vi "Step Response - Air Heater.vi"() -> ()   [LabVIEW 2021]
uses:
  <vilib>/Simulation/Scripting/Companion Diagram/SimConfigNode/SimParams.ctl
  <vilib>/Simulation/Scripting/Companion Diagram/SimConfigNode/_simSolvers.ctl
  <vilib>/Simulation/Implementation/Shared/SIMSCR Execution Mode.ctl
  <vilib>/Simulation/Param Hierarchy/Typedefs/SIMPH Param Control Actions.ctl
  <vilib>/Simulation/Implementation/Shared/NILVSim_ParamChanged.vi
  <vilib>/Simulation/Implementation/Shared/NILVSIM_BeginStep.vi
  <vilib>/Simulation/Implementation/Shared/NILVSim_Manager.vi
  <vilib>/Utility/error.llb/Clear Errors.vi
  <vilib>/Simulation/Implementation/Shared/NILVSim_FinalizeModel.vi
  <vilib>/Simulation/Implementation/Shared/SIM Unbundle Sim Info.vi
  <vilib>/Simulation/Implementation/Shared/NILVSim_Initialize.vi
  <vilib>/Simulation/Utility/Implementation/NILVSim Get Time and IsAcceptedStep.vi
  <vilib>/Simulation/Implementation/Shared/SIMSH Read Queue.vi
  <vilib>/Simulation/Implementation/Shared/NILVSim_GetModelError.vi
  <vilib>/Simulation/Implementation/Shared/SIM Bundle Sim Info.vi
  <vilib>/Simulation/Implementation/XNodeFramework/SimXNode/SimX.xnode
  Model - Air Heater.vi
  <vilib>/Simulation/Scripting/Companion Diagram/SimConfigNode/SimDog.xnode
  <vilib>/Simulation/Implementation/Shared/NI_SIM_Implementation.lvlib
panel:
  in  "T_init [C]":dbl
  in  "T [s]":dbl
  in  "T_delay [s]":dbl
  in  "T_env [C]":dbl
  in  "K [C/V]":dbl
  in  "u [V]":dbl
  in  "Time Step [s]":dbl
  in  "stop":bool
  out "Control chart":dbl(graph)
  out "Temperature Chart":dbl(graph)
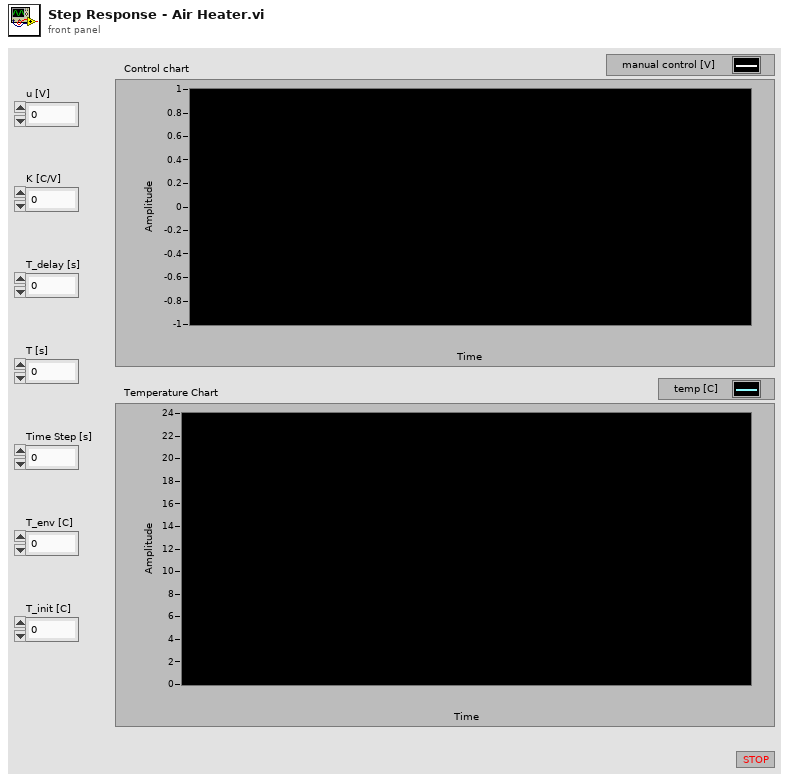
[diagram p1: front panel]
types:
  T1 = enum16{"Simulate to Completion", "Single Time-Step Simulation (Fixed Step Only)"}
  T2 = typedef "SIMSCR Execution Mode.ctl" = enum16{"Simulate to Completion", "Single Time-Step Simulation (Fixed Step Only)"}
  T3 = typedef "SIMPH Param Control Actions.ctl" = enum16{"get params", "set params"}
  T4 = cluster{"SIMSH Sim Time":dbl, "lower limit":dbl, "Divide":cluster{"x/y":dbl}, "Subtract":cluster{"x-y":dbl}, "Transport Delay":cluster{"output":dbl}, "Integrator":cluster{"output":dbl}, "Add":cluster{"x+y":dbl}, "Multiply":cluster{"x*y":dbl}}
  T5 = typedef "SimParams.ctl" = cluster{"Initial Time (s)":dbl, "Final Time (s)":dbl, "Step Size (s)":dbl, "ODE Solver":T6, "Minimum Step Size (s)":dbl, "Maximum Step Size (s)":dbl, "Relative Tolerance":dbl, "Absolute Tolerance":dbl, "Software Timing":bool, "Initial Step Size (s)":dbl, "Automatic Fixed Step Size?":bool, "Automatic Discrete Step Size?":bool, "Discrete Step Size (s)":dbl, "Calculate using Time Step":bool, "Solver Wired?":bool, "Prev.Frm.Expected End":u64, "Prev.Frm.Actual End":u64, "Prev.Frm.Finished Late?":bool, "Prev.Iter.Expected End":u64, "Prev.Iter.Actual End":u64, "Prev.Iter.Finished Late?":bool, "Expected Iteration Start":u64, "Actual Iteration Start":u64, "Expected Frame Start":u64, "Actual Frame Start":u64, "Source Name":string, "Name":string, "Period":i64, "Deadline":i64, "Offset":i64, "Start":i64, "Priority":i32, "Timeout":i32, "Processor":i32, "Mode":enum32{"No Change", "Process missed periods, maintain original phase", "Discard missed periods, maintain original phase", "Process missed periods, ignore original phase", "Discard missed periods, ignore original phase"}, "Wakeup reason":enum32{"Normal", "Aborted", "Asynchronous wakeup", "Timing source error", "Timed loop error", "Timeout"}, "Error":errorcluster, "Source Type":string, "Secondary Source Type":string, "Global End Time":u64, "Global Start Time":u64, "Full Solver Reset":bool, "Execution Mode":T2, "Nan/Inf Check":bool, "Custom Solver Library":string, "Solver Is Variable":bool, "custom solver name":string, "Signal Collection Decimation":u32}
  T6 = typedef "_simSolvers.ctl" = enum16{"Runge-Kutta 1 (Euler)", "Runge-Kutta 2", "Runge-Kutta 3", "Runge-Kutta 4", "Runge-Kutta 23 (variable)", "Runge-Kutta 45 (variable)", "BDF (variable)", "Adams-Moulton (variable)", "Rosenbrock (variable)", "Discrete States Only", "SDIRK 4 (variable)", "Radau 5 (variable)", "Radau 9 (variable)", "Radau 13 (variable)", "Radau [Variable Order] (variable)", "Gear's Method (variable)", "Linearizer", "State Query", "Trim Eval", "Custom Solver"}
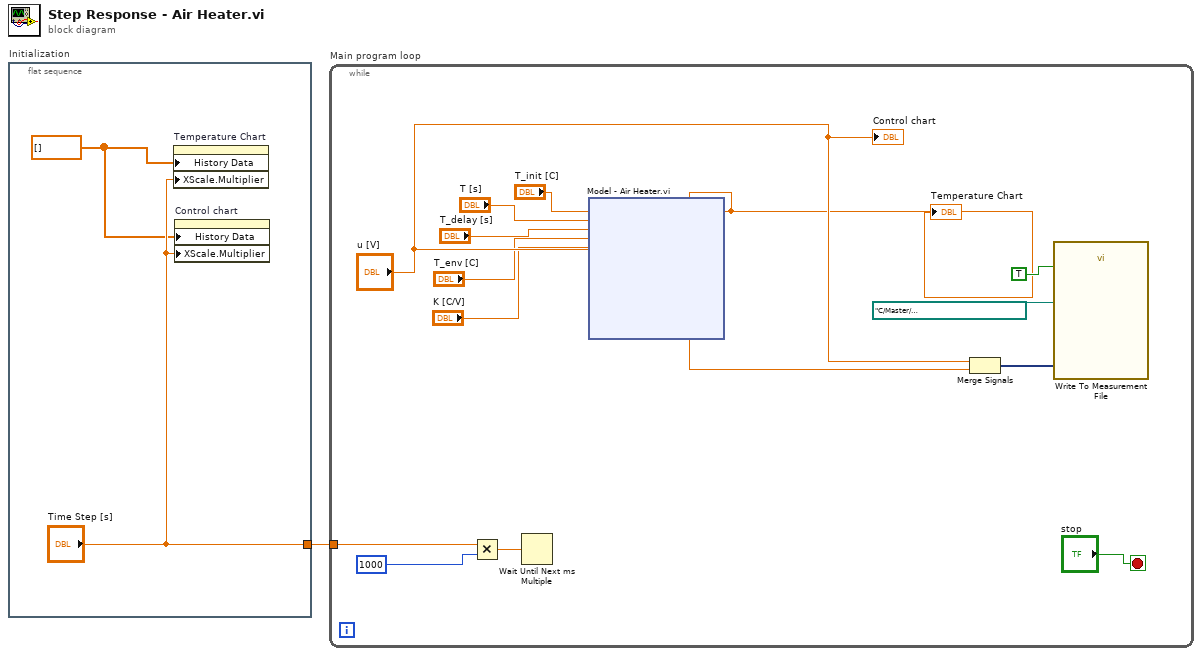
[diagram p0: block diagram]
diagram:
  n1 = flat-sequence "Initialization" {
    tunnel: ["Time Step [s]"] -> w1
    frame #0 {
      w2 = dbl[] [] ("History Data")
      n2 = property on="Temperature Chart" class="WFChart (strict)"("History Data"=w2, "XScale.Multiplier"="Time Step [s]") -> ()  [unwired: 2 in, 2 out]
      n3 = property on="Control chart" class="WFChart (strict)"("History Data"=w2, "XScale.Multiplier"="Time Step [s]") -> ()  [unwired: 2 in, 2 out]
    }
  }
  n4 = while "Main program loop" {
    tunnel: w1 -> [w10]
    stop <- "stop" stop-if-true
    n5 = Multiply(x=w10, y=u32 1000 ("milliseconds to wait")) -> (x*y=w12:dbl)
    n6 = Wait Until Next ms Multiple(millisecond multiple=w12) -> ()  [unwired: 1 out]
    n7 = xnode "Model - Air Heater.vi"("T_init [C]"="T_init [C]", "T [s]"="T [s]", "T_delay [s]"="T_delay [s]", "T_env [C]"="T_env [C]", "K [C/V]"="K [C/V]", "u [V]"="u [V]") -> ("T_out [C]"=w4:dbl)  [unwired: 2 in, 6 out]
    "Temperature Chart" <- w4
    n8 = Merge Signals("u [V]", w4) -> (w14:dynamicdata)
    n9 = call "Write To Measurement File"("Signals"=w14, "Enable"=TRUE, "Filename"=path "C:/Master/Industrial-information-technology/HIL/HIL_Measurements.lvm") -> ()  [unwired: 14 in, 3 out]
    "Control chart" <- "u [V]"
  }
